vi "Polling Control Data From PLC.vi"(7 "Polling Data Input":T1, 8 "error in (no error)":errorcluster, 11 "TCP Network Connection in":refnum<k5>) -> (0 "error out":errorcluster, 1 "Data Read":u8[][](array[numeric]), 2 "PLC Data out":T1, 3 "TCP Network Connection out":refnum<k5>, 4 "Bool Data Valid":bool, 5 "Float Data Valid?":bool[](array[boolean]), 6 "Motor2RatingRPM":u16)   [LabVIEW 2018]
uses:
  Ctls/DisplayIndicator.ctl
  Ctls/MotroConfigData.ctl
  Ctls/MotorConfig.ctl
  Ctls/MagType.ctl
  Siemens S7 TCP v3_3 LV 8_5/Siemens S7 TCP v3_3 LV 8_5/S7 TCP API Library/S7 TCP.lvlib
panel:
  out "Motor1RatingRPM":u16
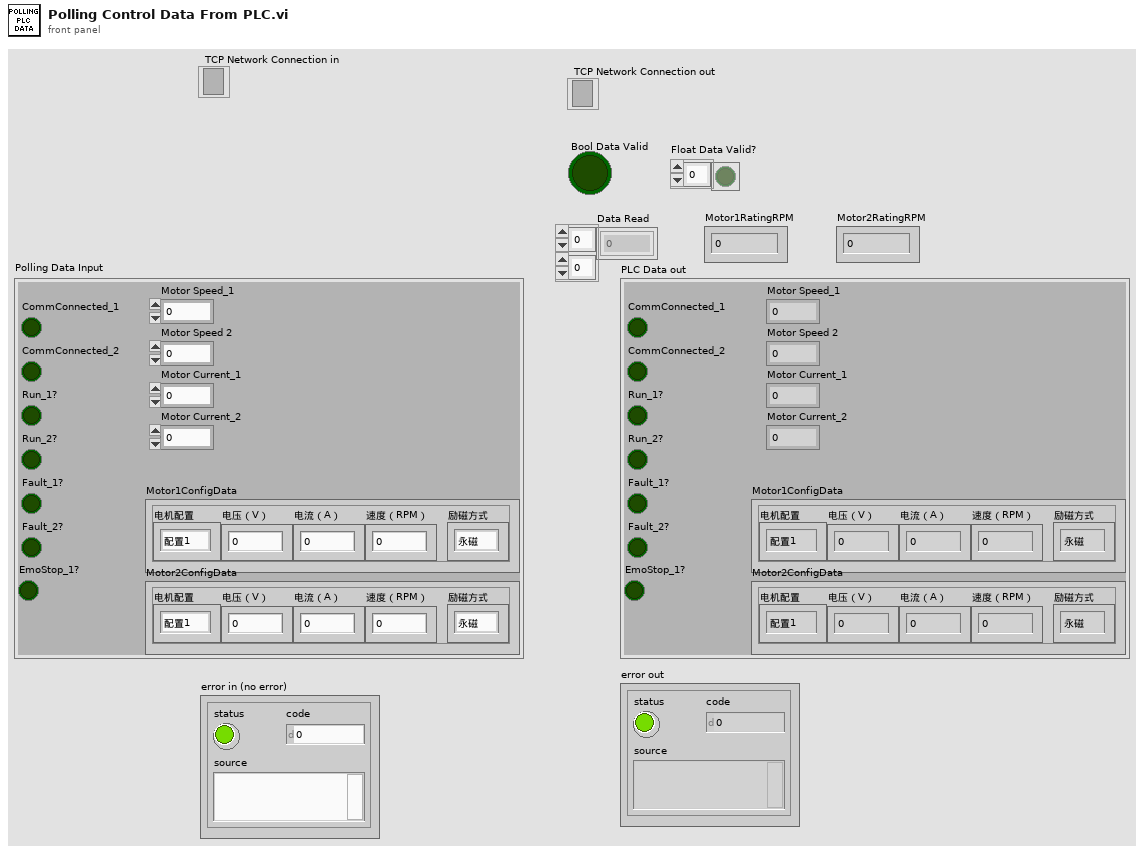
[diagram p1: front panel]
types:
  T1 = typedef "DisplayIndicator.ctl" = cluster{"CommConnected_1":bool, "Run_1?":bool, "Fault_1?":bool, "CommConnected_2":bool, "Run_2?":bool, "Fault_2?":bool, "Motor Speed 2":sgl, "Motor Speed_1":sgl, "Motor Current_1":sgl, "Motor Current_2":sgl, "Motor1ConfigData":T2, "Motor2ConfigData":T2, "EmoStop_1?":bool}
  T2 = typedef "MotroConfigData.ctl" = cluster{"电机配置":T3, "电压（V）":dbl, "电流（A）":dbl, "速度（RPM）":dbl, "励磁方式":T4}
  T3 = typedef "MotorConfig.ctl" = enum16{"配置1", "配置2", "配置3", "配置4"}
  T4 = typedef "MagType.ctl" = enum16{"永磁", "励磁"}
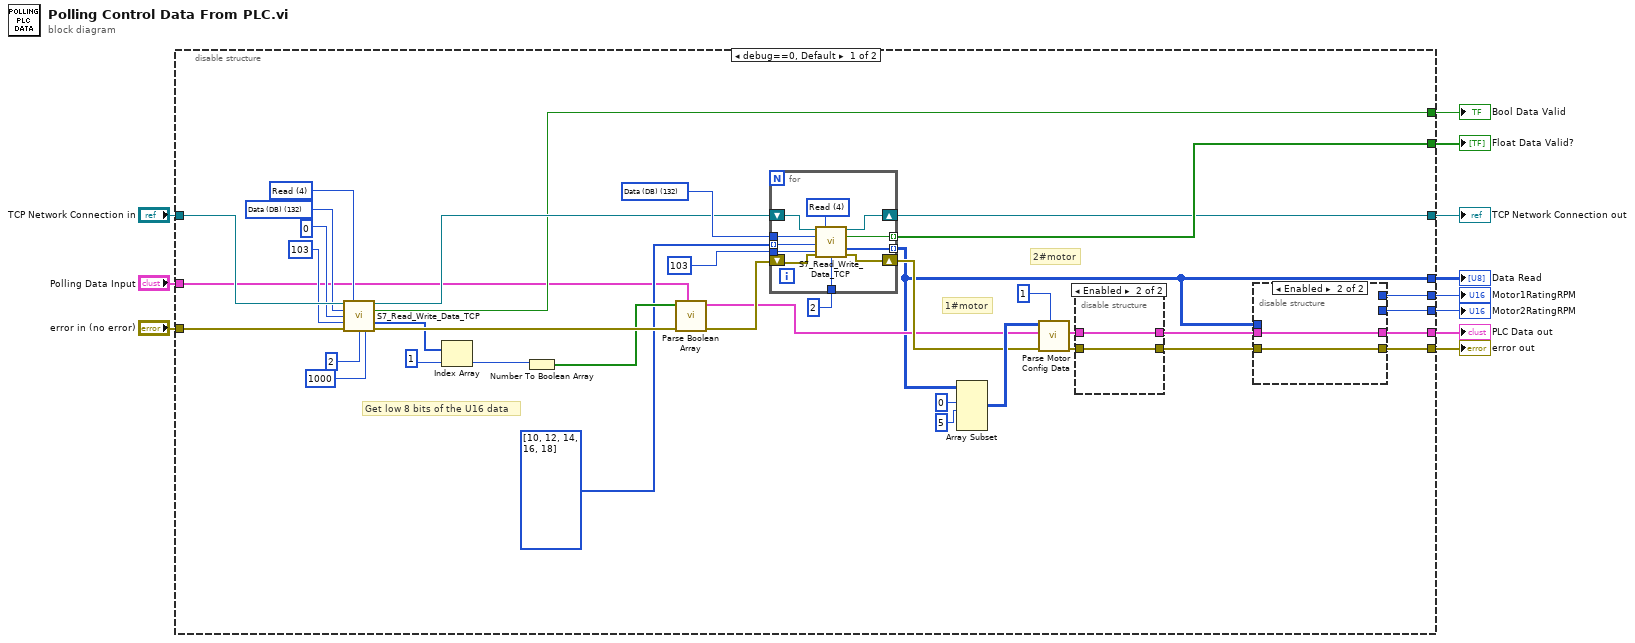
[diagram p0: block diagram]
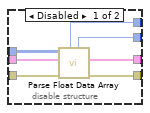
[diagram p2: hidden frame]
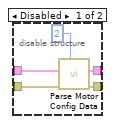
[diagram p3: hidden frame]
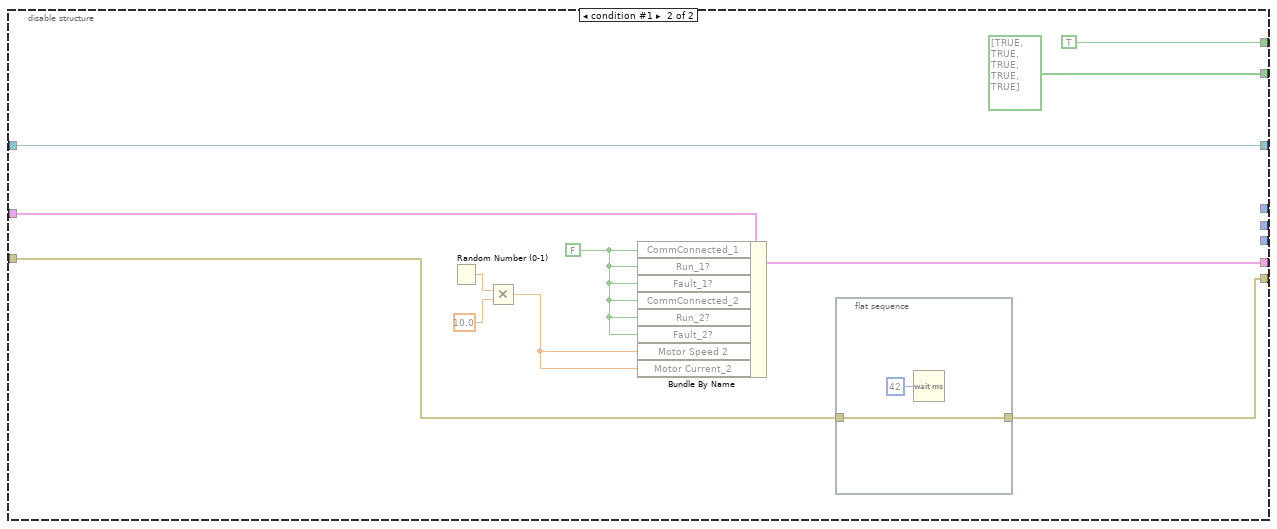
[diagram p4: hidden frame]
diagram:
  n1 = disable-structure shown="debug==0, Default" {
    disable-tunnel: [w49 w85] -> w11
    disable-tunnel: [w48 w78] -> w10
    disable-tunnel: [w18 _] -> w9
    disable-tunnel: [w47 bool[] [TRUE, TRUE, TRUE, TRUE, TRUE]] -> w8
    disable-tunnel: [w43 w88] -> w7
    disable-tunnel: [w40 TRUE ("Data Valid")] -> w6
    disable-tunnel: "TCP Network Connection in" -> [w39 w88]
    disable-tunnel: "error in (no error)" -> [w38 w79]
    disable-tunnel: [w16 _] -> w3
    disable-tunnel: [w15 _] -> w2
    disable-tunnel: "Polling Data Input" -> [w12 w80]
    frame condition #0 (active) {
      w32 = u8 132 items=["I/O (P)"=128, "Input (I)"=129, "Output (Q)"=130, "Bit Memory (M)"=131, "Data (DB)"=132, "Instance Data (DI)"=133, "Local Data (L)"=134, "Predecessor Local Data (VL)"=135] ("Address Areas")
      w31 = u8 4 items=["Read"=4, "Write"=5] ("Read / Write")
      w42 = u8 132 items=["I/O (P)"=128, "Input (I)"=129, "Output (Q)"=130, "Bit Memory (M)"=131, "Data (DB)"=132, "Instance Data (DI)"=133, "Local Data (L)"=134, "Predecessor Local Data (VL)"=135] ("Address Areas")
      # "2#motor"
      # "1#motor"
      # "Get low 8 bits of the U16 data"
      n2 = call "S7_Read_Write_Data_TCP.vi"("TCP Connection Ref"=w39, "Read / Write"=w31, "Address Areas"=w32, "Start Address (bytes)"=u32 0, "Data Block #"=u16 103, "error in"=w38, "Length (bytes)"=u16 2, "Timeout"=u32 1000) -> ("TCP Connection Ref Out"=w41:refnum<k5>, "Data Valid"=w40:bool, "Data Read"=w30:u8[], "error out"=w37:errorcluster)  [unwired: 2 in, 2 out]
      n3 = Index Array(array=w30, index=1) -> (element=w28:u8)
      n4 = Number To Boolean Array(number=w28) -> (Boolean array=w36:bool[])
      n5 = call "Parse Boolean Array.vi"("Polling Data Input"=w12, "error in (no error)"=w37, "Bool Array Input"=w36) -> ("error out"=w45:errorcluster, "output cluster"=w21:T1)  [unwired: 7 in]
      n6 = for {
        tunnel: w42 -> [w76]
        tunnel: u16 103 ("Data Block #") -> [w73]
        tunnel: u32[] [10, 12, 14, 16, 18] -> [w72] mode=indexing
        tunnel: u16 2 ("Length (bytes)") -> [w71]
        tunnel: [w70] -> w47 mode=indexing
        tunnel: [w69] -> w18 mode=indexing
        shift-right: [w67] -> w24
        shift-left: w45 -> [w68]
        shift-right: [w74] -> w43
        shift-left: w41 -> [w77]
        w75 = u8 4 items=["Read"=4, "Write"=5] ("Read / Write")
        n7 = call "S7_Read_Write_Data_TCP.vi"("TCP Connection Ref"=w77, "Read / Write"=w75, "Address Areas"=w76, "Start Address (bytes)"=w72, "Data Block #"=w73, "error in"=w68, "Length (bytes)"=w71) -> ("TCP Connection Ref Out"=w74:refnum<k5>, "Data Valid"=w70:bool, "Data Read"=w69:u8[], "error out"=w67:errorcluster)  [unwired: 3 in, 2 out]
      }
      n8 = Array Subset(array=w18, index (row)=0 ("index"), length (row)=5 ("length")) -> (w25:u8[][])  [unwired: 2 in]
      n9 = call "Parse Motor Config Data.vi"("Motor NO"=u8 1, "error in (no error)"=w24, "PLC Data in"=w21, "Data Read"=w25) -> ("error out"=w23:errorcluster, "PLC Data out"=w20:T1)  [unwired: 6 in]
      n10 = disable-structure shown="Enabled" {
        disable-tunnel: w23 -> [w63 w65]
        disable-tunnel: [w62 w65] -> w22
        disable-tunnel: w20 -> [w61 w66]
        disable-tunnel: [w60 w66] -> w19
        frame Disabled {
          n11 = call "Parse Motor Config Data.vi"("Motor NO"=u8 2, "error in (no error)"=w63, "PLC Data in"=w61) -> ("error out"=w62:errorcluster, "PLC Data out"=w60:T1, "Data Read"=w64:u8[][])  [unwired: 6 in]
        }
        frame Enabled {
        }
      }
      n12 = disable-structure shown="Enabled" {
        disable-tunnel: [w56 w58] -> w49
        disable-tunnel: [w55 w57] -> w48
        disable-tunnel: w22 -> [w54 w57]
        disable-tunnel: w19 -> [w53 w58]
        disable-tunnel: w18 -> [w52 _]
        disable-tunnel: [w51 _] -> w16
        disable-tunnel: [w50 _] -> w15
        frame Disabled {
          n13 = call "Parse Float Data Array.vi"("error in (no error)"=w54, "PLC Data in"=w53, "Data Read"=w52) -> ("error out"=w55:errorcluster, "PLC Data out"=w56:T1, "Motor2RatingRPM"=w50:u16, "Motor1RatingRPM"=w51:u16)  [unwired: 5 in]
        }
        frame Enabled {
        }
      }
    }
    frame condition #1 {
      w84 = FALSE ("CommConnected_1")
      n14 = Random Number (0-1)() -> (number: 0 to 1=w83:dbl)
      n15 = Multiply(x=w83, y=10.0) -> (x*y=w81:dbl)
      n16 = Bundle By Name(cluster=w80, "CommConnected_1"=w84, "Run_1?"=w84, "Fault_1?"=w84, "CommConnected_2"=w84, "Run_2?"=w84, "Fault_2?"=w84, "Motor Speed 2"=w81, "Motor Current_2"=w81) -> (w85:T1)
      n17 = flat-sequence {
        tunnel: w79 -> [w89]
        tunnel: [w89] -> w78
        frame #0 {
          n18 = Wait (ms)(milliseconds to wait=u32 42) -> ()  [unwired: 1 out]
        }
      }
    }
  }
  "Bool Data Valid" <- w6
  "Float Data Valid?" <- w8
  "Data Read" <- w9
  "PLC Data out" <- w11
  "error out" <- w10
  "TCP Network Connection out" <- w7
  "Motor1RatingRPM" <- w3
  "Motor2RatingRPM" <- w2
